vi "midi-track.add.vi"(8 "error in (no error)":errorcluster, 9 "Track Events":refnum<class "midi-file-event.lvclass">[](array[class]), 10 "Track Number":i32, 11 "midi-file-events in":refnum<class "midi-file-events.lvclass">) -> (0 "error out":errorcluster, 3 "midi-file-events out":refnum<class "midi-file-events.lvclass">)   [LabVIEW 2020, in "midi-file-events.lvclass"]
uses:
  midi-file-events.lvclass
  midi-file-event/midi-file-event.lvclass
  midi-file-events.lvclass/midi-file-events.ctl
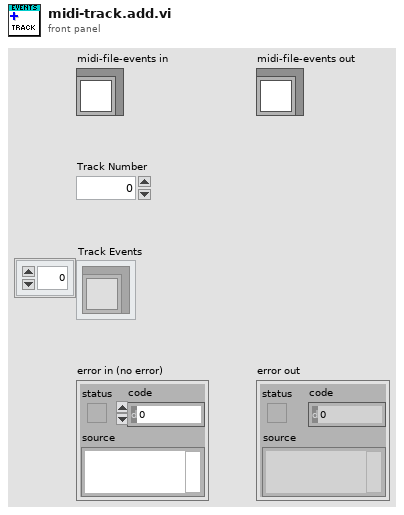
[diagram p1: front panel]
types:
  T1 = map{i32, refnum<class "midi-file-event.lvclass">[]}
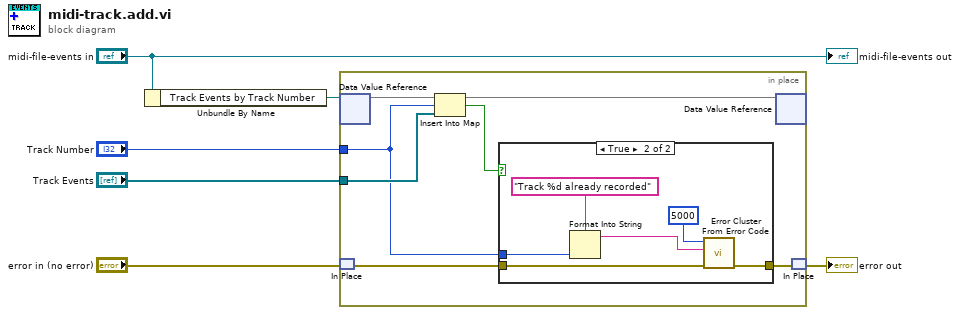
[diagram p0: block diagram]
diagram:
  n1 = Unbundle By Name("midi-file-events in") -> ("Track Events by Track Number"=w6:refnum<data-value>)
  n2 = in-place {
    in-place-border: "Track Number" -> [w9]
    in-place-border: "Track Events" -> [w12]
    n3 = in-place-dvr #1(w6) -> (w13:T1)  [unwired: 1 out]
    n4 = in-place-match #2("error in (no error)") -> (w8:errorcluster)
    n5 = Insert Into Map(map in=w13, key=w9, value=w12) -> (map out=w11:T1, key already included?=w10:bool)  [unwired: 1 out]
    n6 = case shown="True" w10 {
      tunnel: w9 -> [_ w19]
      tunnel: w8 -> [w14 w16]
      tunnel: [w14 w15] -> w7
      frame False {
      }
      frame True {
        n7 = Format Into String(format string="Track %d already recorded", w19) -> (resulting string=w17:string)  [unwired: 2 in, 1 out]
        n8 = call <vilib>:"Error Cluster From Error Code.vi"("error in (no error)"=w16, "error message (\"\")"=w17, "error code (0)"=5000) -> ("error out"=w15:errorcluster)  [unwired: 6 in]
      }
    }
    n9 = in-place-dvr #1(w11) -> ()  [unwired: 2 out]
    n10 = in-place-match #2(w7) -> (→"error out":errorcluster)
  }
  "midi-file-events out" <- "midi-file-events in"
